vi "XY Graph Get Plot.vi"(8 "error in (no error)":errorcluster, 10 "Plot Index (-1: last)":i32=-1, 11 "XYGraph in":T2) -> (0 "error out":errorcluster, 1 "Plot Name":string, 2 "Plot Data":T1, 3 "XYGraph out":T2, 5 "Graph Name":string)   [LabVIEW 2021, in "XY Graph Add-Ons.lvlib"]
uses:
  XY Graph Add-Ons.lvlib
  XY Graph Refnum.ctl
  XY Graph Plot Data.ctl
  Arrays/Arrays.lvlib
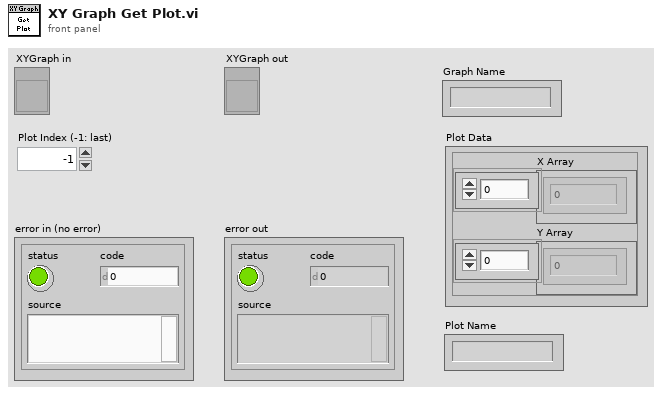
[diagram p1: front panel]
types:
  T1 = typedef "XY Graph Add-Ons.lvlib/XY Graph Plot Data.ctl" = cluster{"X Array":dbl[], "Y Array":dbl[]}
  T2 = typedef "XY Graph Add-Ons.lvlib/XY Graph Refnum.ctl" = refnum<vi>
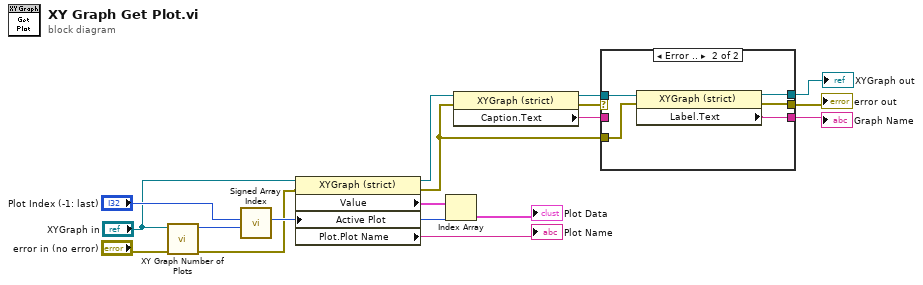
[diagram p0: block diagram]
diagram:
  n1 = call "XY Graph Number of Plots.vi"("Error In"="error in (no error)", "XYGraph in"="XYGraph in") -> ("Error Out"=w11:errorcluster, "# Plots"=w16:i32)  [unwired: 8 in]
  n2 = call "Signed Array Index.vi"("Array Size"=w16, "Array Index in"="Plot Index (-1: last)") -> ("Array Index out"=w13:i32)  [unwired: 9 in]
  n3 = property class="XYGraph (strict)"(reference="XYGraph in", error in=w11, "Active Plot"=w13) -> (reference out=w8:T2, error out=w3:errorcluster, "Value"=w14:cluster{"X Array":dbl[], "Y Array":dbl[]}[], "Plot.Plot Name"=→"Plot Name":string)
  n4 = Index Array(array=w14, index=w13) -> (element=→"Plot Data":cluster{"X Array":dbl[], "Y Array":dbl[]})
  n5 = property class="XYGraph (strict)"(reference=w8, error in=w3) -> (reference out=w2:T2, error out=w7:errorcluster, "Caption.Text"=w6:string)
  n6 = case shown="Error .." w7 {
    selector: w7 -> [w19 _]
    tunnel: w6 -> [w20 _]
    tunnel: [w20 w22] -> w5
    tunnel: [w19 w23] -> w4
    tunnel: w2 -> [w18 w25]
    tunnel: w3 -> [_ w24]
    tunnel: [w18 w21] -> w1
    frame No Error {
    }
    frame Error {
      n7 = property class="XYGraph (strict)"(reference=w25, error in=w24) -> (reference out=w21:T2, error out=w23:errorcluster, "Label.Text"=w22:string)
    }
  }
  "XYGraph out" <- w1
  "error out" <- w4
  "Graph Name" <- w5
